vi "Instrument Type ID.vi"() -> (1 "instrument type id":string="niSE")   [LabVIEW 2021, in "NI Session Management niSE.lvlib"]
uses:
  NI Session Management niSE.lvlib
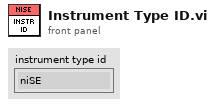
[diagram p1: front panel]
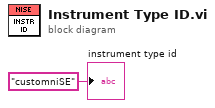
[diagram p0: block diagram]
diagram:
  "instrument type id" <- "customniSE" ("instrument type id")
